vi "ShowAll.vi"(0 "reference in":refnum<class "Customers.lvclass">, 5 "error in (no error)":errorcluster) -> (14 "reference out":refnum<class "Customers.lvclass">, 19 "error out":errorcluster)   [LabVIEW 2020, in "Customers.lvclass"]
uses:
  Customers.lvclass
  C:/Projects/OpenGDS_DesignPatterns/Bridge1/CustomersBase_class/CustomersBase.lvclass
  CustomersBase_class/CustomersBase.lvclass
  DataObject_class/DataObject.lvclass
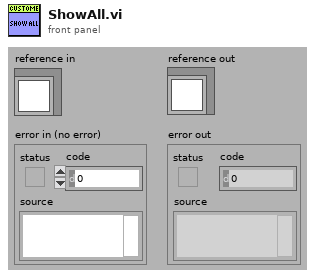
[diagram p1: front panel]
types:
  T1 = typedef "CustomersBase.lvclass/ObjectAttributes.ctl" = cluster{"_dataObject":refnum<class "DataObject.lvclass">, "Group":string}
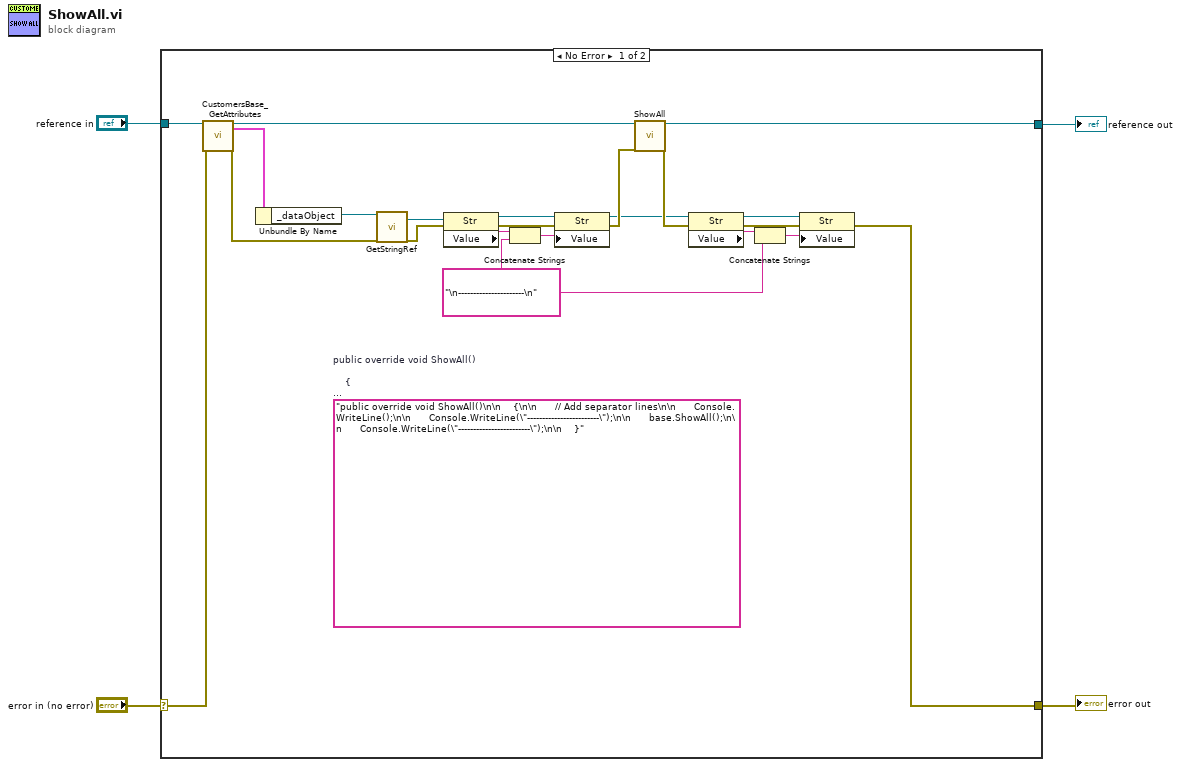
[diagram p0: block diagram]
diagram:
  n1 = case shown="No Error" "error in (no error)" {
    selector: "error in (no error)" -> [w25 w28]
    tunnel: [w7 w28] -> w3
    tunnel: [w19 w27] -> w1
    tunnel: "reference in" -> [w26 w27]
    frame No Error {
      w5 = "\n----------------------\n" ("format string")
      (unwired) "public override void ShowAll()\n\n    {\n\n      // Add separator lines\n\n      Console.WriteLine();\n\n      Console.WriteLine(\"------------------------\");\n\n      base.ShowAll();\n\n      Console.WriteLine(\"------------------------\");\n\n    }"  # public override void ShowAll()      {        // Add separator lines        Console.WriteLine();        Console.WriteLine("------------------------");        base.ShowAll();        Console.WriteLine("------------------------");      }
      n2 = call "CustomersBase_GetAttributes.vi"("reference in"=w26, "error in (no error)"=w25) -> ("reference out"=w20:refnum<class "Customers.lvclass">, "Data"=w24:T1, "error out"=w13:errorcluster)  [unwired: 14 in, 1 out]
      n3 = Unbundle By Name(w24) -> ("_dataObject"=w23:refnum<class "DataObject.lvclass">)
      n4 = call-dynamic "GetStringRef.vi"("reference in"=w23, "error in (no error)"=w13) -> ("StringRef"=w22:refnum<vi>, "error out"=w14:errorcluster)  [unwired: 15 in, 1 out]
      n5 = property class="Str"(reference=w22, error in=w14) -> (reference out=w21:refnum<vi>, error out=w15:errorcluster, "Value"=w18:string)
      n6 = Concatenate Strings(w18, w5) -> (w17:string)
      n7 = property class="Str"(reference=w21, error in=w15, "Value"=w17) -> (reference out=w6:refnum<vi>, error out=w16:errorcluster)
      n8 = call-parent "ShowAll.vi"("reference in"=w20, "error in (no error)"=w16) -> ("reference out"=w19:refnum<class "Customers.lvclass">, "error out"=w8:errorcluster)  [unwired: 16 in]
      n9 = property class="Str"(reference=w6, error in=w8) -> (reference out=w9:refnum<vi>, error out=w12:errorcluster, "Value"=w10:string)
      n10 = Concatenate Strings(w10, w5) -> (w11:string)
      n11 = property class="Str"(reference=w9, error in=w12, "Value"=w11) -> (error out=w7:errorcluster)  [unwired: 1 out]
    }
    frame Error {
    }
  }
  "error out" <- w3
  "reference out" <- w1
